vi "Move Conveyer Belt.vi"(6 "Frisbee States":T1, 7 "Enable Stack":bool, 8 "frisbee counter":i16, 9 "Suck":bool) -> (0 "move conveyer belt":bool)   [LabVIEW 2012]
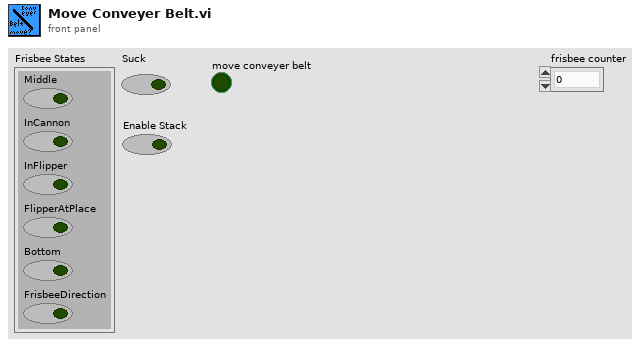
[diagram p1: front panel]
types:
  T1 = cluster{"Middle":bool, "InCannon":bool, "InFlipper":bool, "FlipperAtPlace":bool, "Bottom":bool, "FrisbeeDirection":bool}
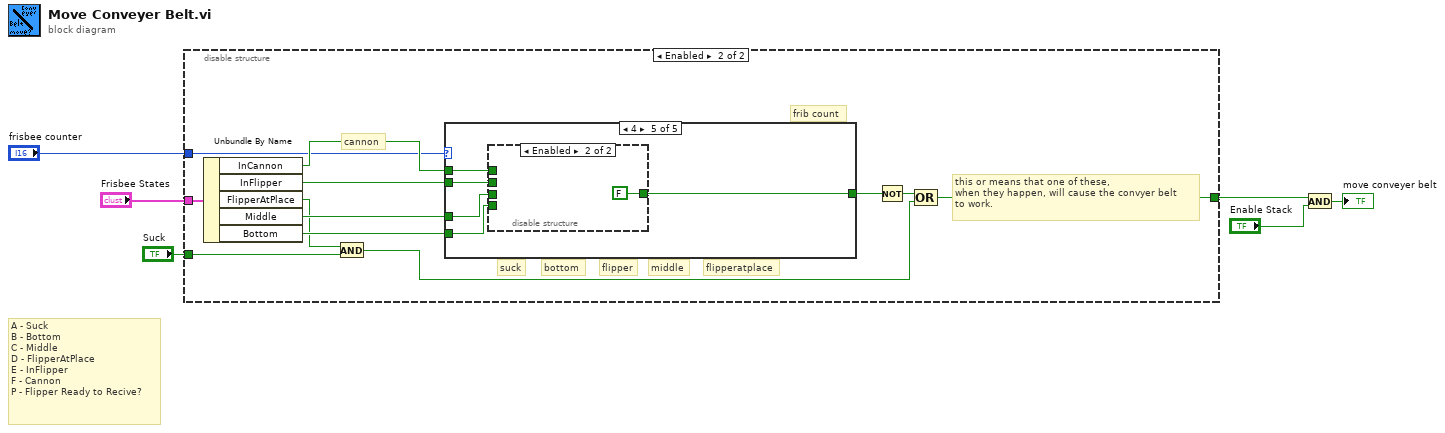
[diagram p0: block diagram]
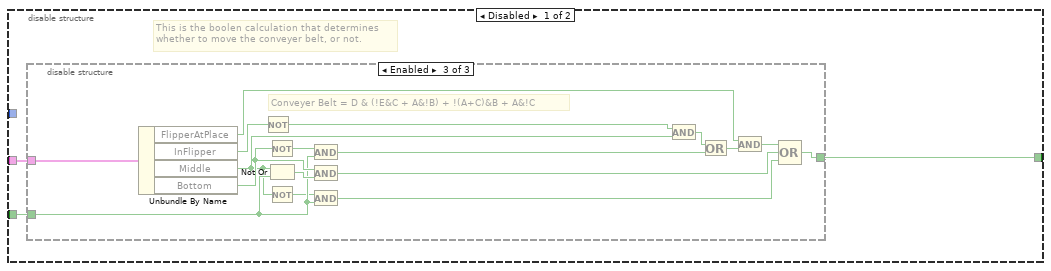
[diagram p2: hidden frame]
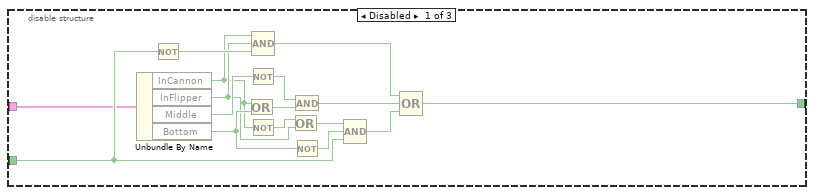
[diagram p3: hidden frame]
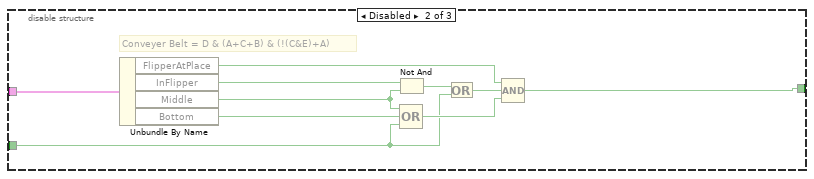
[diagram p4: hidden frame]
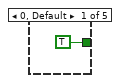
[diagram p5: hidden frame]
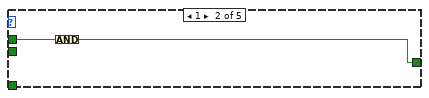
[diagram p6: hidden frame]
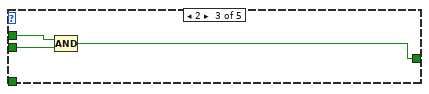
[diagram p7: hidden frame]
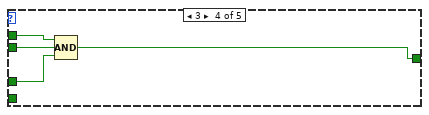
[diagram p8: hidden frame]
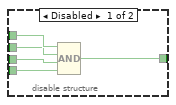
[diagram p9: hidden frame]
diagram:
  # "A - Suck\nB - Bottom\nC - Middle\nD - FlipperAtPlace\nE - InFlipper\nF - Cannon\nP - Flipper Ready to Recive?"
  n1 = disable-structure shown="Enabled" {
    disable-tunnel: "Frisbee States" -> [w9 w57]
    disable-tunnel: "Suck" -> [w8 w54]
    disable-tunnel: "frisbee counter" -> [_ w58]
    disable-tunnel: [w7 w56] -> w1
    frame Disabled {
      # "This is the boolen calculation that determines\nwhether to move the conveyer belt, or not."
      n2 = disable-structure shown="Enabled" {
        disable-tunnel: [w12 w33 w36] -> w7
        disable-tunnel: w8 -> [w11 w27 w40]
        disable-tunnel: w9 -> [w10 w35 w52]
        frame Disabled {
          n3 = Unbundle By Name(w10) -> ("InCannon"=w14:bool, "InFlipper"=w15:bool, "Middle"=w22:bool, "Bottom"=w19:bool)
          n4 = Not(x=w11) -> (.not. x?=w16:bool)
          n5 = Or(x=w14, y=w19) -> (x .or. y?=w20:bool)
          n6 = Not(x=w22) -> (.not. x?=w21:bool)
          n7 = Not(x=w14) -> (.not. x?=w24:bool)
          n8 = Compound Arithmetic op=AND(w14, w15, w16) -> (w13:bool)
          n9 = Or(x=w24, y=w15) -> (x .or. y?=w23:bool)
          n10 = And(x=w21, y=w20) -> (x .and. y?=w18:bool)
          n11 = Not(x=w19) -> (.not. x?=w25:bool)
          n12 = Compound Arithmetic op=AND(w23, w25, w11) -> (w17:bool)
          n13 = Compound Arithmetic op=OR(w13, w18, w17) -> (w12:bool)
        }
        frame Disabled {
          # "Conveyer Belt = D & (A+C+B) & (!(C&E)+A)"
          n14 = Unbundle By Name(w35) -> ("FlipperAtPlace"=w32:bool, "InFlipper"=w30:bool, "Middle"=w29:bool, "Bottom"=w34:bool)
          n15 = Not And(1:w29, 2:w30) -> (0:w28:bool)
          n16 = Compound Arithmetic op=OR(w29, w34, w27) -> (w31:bool)
          n17 = Or(x=w28, y=w27) -> (x .or. y?=w26:bool)
          n18 = Compound Arithmetic op=AND(w32, w26, w31) -> (w33:bool)
        }
        frame Enabled {
          # "Conveyer Belt = D & (!E&C + A&!B) + !(A+C)&B + A&!C"
          n19 = Unbundle By Name(w52) -> ("FlipperAtPlace"=w45:bool, "InFlipper"=w51:bool, "Middle"=w38:bool, "Bottom"=w42:bool)
          n20 = Not(x=w51) -> (.not. x?=w50:bool)
          n21 = Not(x=w42) -> (.not. x?=w47:bool)
          n22 = Not Or(1:w40, 2:w38) -> (0:w43:bool)
          n23 = Not(x=w38) -> (.not. x?=w39:bool)
          n24 = And(x=w47, y=w40) -> (x .and. y?=w48:bool)
          n25 = And(x=w42, y=w43) -> (x .and. y?=w41:bool)
          n26 = And(x=w39, y=w40) -> (x .and. y?=w37:bool)
          n27 = And(x=w50, y=w38) -> (x .and. y?=w49:bool)
          n28 = Or(x=w49, y=w48) -> (x .or. y?=w46:bool)
          n29 = And(x=w45, y=w46) -> (x .and. y?=w44:bool)
          n30 = Compound Arithmetic op=OR(w44, w41, w37) -> (w36:bool)
        }
      }
    }
    frame Enabled {
      # "bottom"
      # "middle"
      # "flipperatplace"
      # "flipper"
      # "cannon"
      # "frib count"
      # "suck"
      # "this or means that one of these, \nwhen they happen, will cause the convyer belt\nto work."
      n31 = Unbundle By Name(w57) -> ("InCannon"=w59:bool, "InFlipper"=w60:bool, "FlipperAtPlace"=w55:bool, "Middle"=w62:bool, "Bottom"=w63:bool)
      n32 = And(x=w55, y=w54) -> (x .and. y?=w53:bool)
      n33 = case shown="4" w58 {
        tunnel: w59 -> [_ w67 w69 w72 w79]
        tunnel: w60 -> [_ _ w70 w73 w78]
        tunnel: [TRUE w66 w68 w71 w75] -> w61
        tunnel: w62 -> [_ _ _ w74 w77]
        tunnel: w63 -> [_ _ _ _ w76]
        frame 0, Default {
        }
        frame 1 {
          n34 = Compound Arithmetic op=AND(w67) -> (w66:bool)
        }
        frame 2 {
          n35 = Compound Arithmetic op=AND(w69, w70) -> (w68:bool)
        }
        frame 3 {
          n36 = Compound Arithmetic op=AND(w72, w73, w74) -> (w71:bool)
        }
        frame 4 {
          n37 = disable-structure shown="Enabled" {
            disable-tunnel: w79 -> [w84 _]
            disable-tunnel: w78 -> [w83 _]
            disable-tunnel: w77 -> [w82 _]
            disable-tunnel: w76 -> [w81 _]
            disable-tunnel: [w80 FALSE] -> w75
            frame Disabled {
              n38 = Compound Arithmetic op=AND(w84, w83, w82, w81) -> (w80:bool)
            }
            frame Enabled {
            }
          }
        }
      }
      n39 = Not(x=w61) -> (.not. x?=w64:bool)
      n40 = Compound Arithmetic op=OR(w64, w53) -> (w56:bool)
    }
  }
  n41 = And(x=w1, y="Enable Stack") -> (x .and. y?=→"move conveyer belt":bool)
